vi "Open.vi"(8 "error in (no error)":errorcluster caption="entrée d'erreur (pas d'erreur)", 11 "Class Printer_CAB en entrée":refnum<class "Class Printer_TSC.lvclass">) -> (0 "error out":errorcluster caption="sortie d'erreur", 3 "Class Printer_CAB en sortie":refnum<class "Class Printer_TSC.lvclass">)   [LabVIEW 2020, in "Library Instrument & Equipement.lvlib" / "Library Printer.lvlib" / "Class Printer_TSC.lvclass"]
uses:
  Class Printer_TSC.lvclass
  C:/Users/ngarcin/OneDrive - Altyor/Standard TB/Class/Printer/Printer (Default)/Class Printer (Default).lvclass
  Printer (Default)/Class Printer (Default).lvclass
  Class Printer_TSC.lvclass/Class Printer_TSC.ctl
  TSCLIB/TSCLIB.lvlib
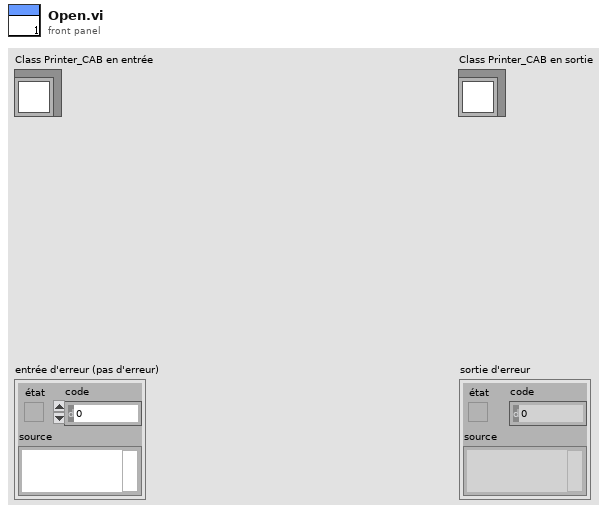
[diagram p1: front panel]
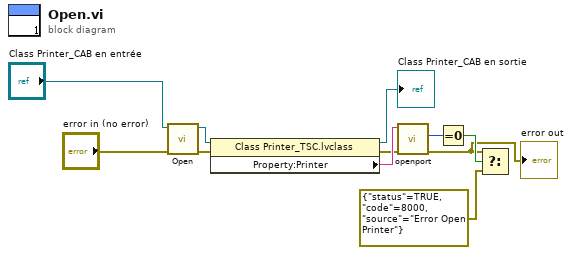
[diagram p0: block diagram]
diagram:
  n1 = call-parent "Open.vi"("error in (no error)"="error in (no error)", "Class Printer (Default) en entrée"="Class Printer_CAB en entrée") -> ("error out"=w7:errorcluster, "Class Printer (Default) en sortie"=w8:refnum<class "Class Printer_TSC.lvclass">)  [unwired: 8 in]
  n2 = property class="Class Printer_TSC.lvclass"(reference=w8, error in=w7) -> (reference out=→"Class Printer_CAB en sortie":refnum<class "Class Printer_TSC.lvclass">, error out=w6:errorcluster, "Property:Printer"=w9:string)
  n3 = call "openport.vi"("error in (no error)"=w6, "para0"=w9) -> ("error out"=w1:errorcluster, "function return"=w5:i32)  [unwired: 7 in, 1 out]
  "error out" <- w1
  n4 = Equal To 0?(x=w5) -> (x = 0?=w4:bool)
  n5 = Select(t=w1, s=w4, f=errorcluster {"status"=TRUE, "code"=8000, "source"="Error Open Printer"} ("cas vrai")) -> ()  [unwired: 1 out]
